vi "LVClass_Camera get Parameter Boolean.vi"(0 "Camera in":refnum<class "Camera.lvclass">, 7 "parameter_name":string, 11 "error in (no error)":errorcluster) -> (4 "Camera out":refnum<class "Camera.lvclass">, 8 "value":bool, 15 "error out":errorcluster)   [LabVIEW 2020, in "Camera.lvclass"]
doc: "Camera parameter getter for parameter of type boolean.\n\n--------------------------------------------------------------------------------\n\n<B>CameraIn </B> : Camera object.\n<B>CameraOut </B> : Camera object.\n<B>parameter_name </B> : Name of the parameter.\n<B>value </B> : Value of the parameter.\n<B>ErrorIn </B> : Error\n<B>ErrorOut </B> : Error\n\n--------------------------------------------------------------------------------"
uses:
  Camera.lvclass
  Camera.lvclass/Camera.ctl
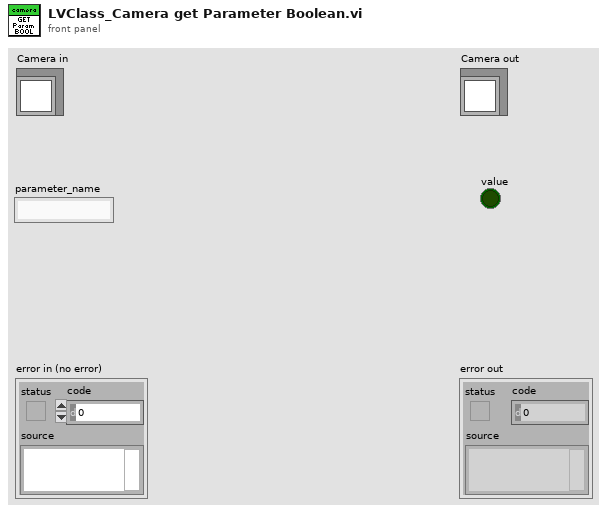
[diagram p1: front panel]
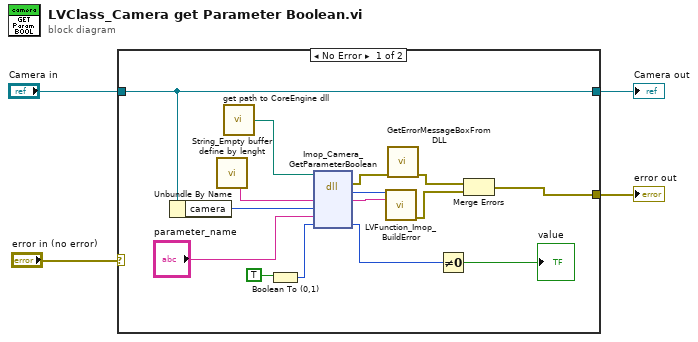
[diagram p0: block diagram]
diagram:
  n1 = case shown="No Error" "error in (no error)" {
    selector: "error in (no error)" -> [_ w21]
    tunnel: [w5 w21] -> w3
    tunnel: [w16 w20] -> w1
    tunnel: "Camera in" -> [w16 w20]
    frame No Error {
      n2 = Unbundle By Name(w16) -> ("camera"=w17:i32)
      n3 = call "String_Empty buffer define by lenght.vi"() -> ("Empty buffer"=w12:string)  [unwired: 1 in]
      n4 = call "get path to CoreEngine dll.vi"() -> ("path to c_interface_vc100.dll"=w15:path)  [unwired: 12 in, 3 out]
      n5 = Boolean To (0,1)(Boolean=TRUE) -> (0, 1=w8:i16)
      n6 = dll-call lib="D:/2_trunk/Soft_haso/ImOpCoreEngine4_LV2011/DLLs/ImopEngine4_vc100.dll" fn="Imop_Camera_GetParameterBoolean"(path in=w15, "message"=w12, "camera"=w17, "parameter_name"="parameter_name", "value"=w8) -> (error out=w14:errorcluster, "return type"=w19:i32, "message"=w18:string, "value"=w10:u8)  [unwired: 4 in, 1 out]
      n7 = call "LVFunction_Imop_BuildError.vi"("code"=w19, "String to Prepend to source (\"\")"=w18) -> ("error out"=w6:errorcluster)  [unwired: 13 in]
      n8 = call "GetErrorMessageBoxFromDLL.vi"("error IN"=w14) -> ("error OUT"=w7:errorcluster)  [unwired: 10 in]
      n9 = Not Equal To 0?(x=w10) -> (x != 0?=→"value":bool)
      n10 = Merge Errors(w7, w6) -> (w5:errorcluster)
    }
    frame Error {
    }
  }
  "error out" <- w3
  "Camera out" <- w1
